vi "Averager Compute with Image.vi"(8 "error in (no error)":errorcluster, 9 "Grayscale Image":T1, 10 "Data":dbl[](array[numeric]), 11 "Roughness Averager in":refnum<class "Roughness Averager.lvclass">) -> (0 "error out":errorcluster, 3 "Roughness Averager out":refnum<class "Roughness Averager.lvclass">)   [LabVIEW 2018, in "Roughness Averager.lvclass"]
uses:
  Roughness Averager.lvclass
  <vilib>/vision/Image Controls.llb/IMAQ Image.ctl
  Roughness Averager.lvclass/Roughness Averager.ctl
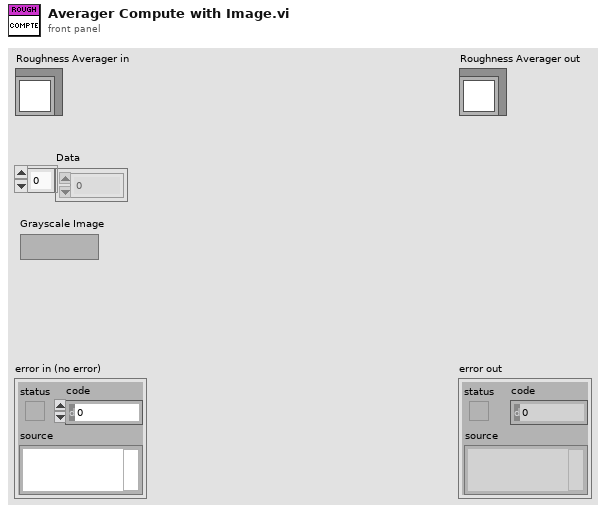
[diagram p1: front panel]
types:
  T1 = typedef "IMAQ Image.ctl" = refnum<image>
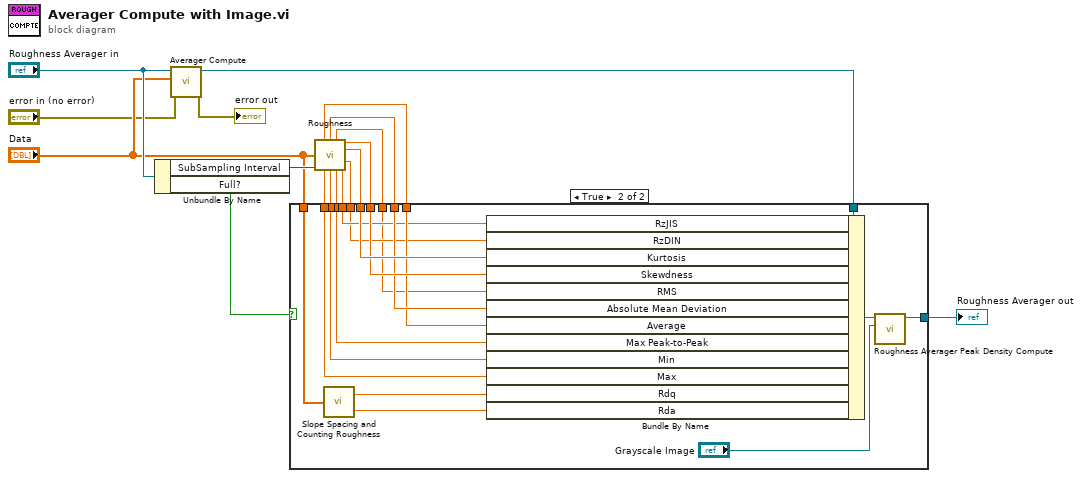
[diagram p0: block diagram]
diagram:
  n1 = Unbundle By Name("Roughness Averager in") -> ("SubSampling Interval"=w18:i32, "Full?"=w6:bool)
  n2 = call-dynamic "Averager Compute.vi"("error in (no error)"="error in (no error)", "Data"="Data", "Roughness Averager in"="Roughness Averager in") -> ("error out"=→"error out":errorcluster, "Roughness Averager out"=w1:refnum<class "Roughness Averager.lvclass">)  [unwired: 7 in]
  n3 = call "Roughness.vi"("Data"="Data", "Sub Sampling Interval (10)"=w18) -> ("Mean"=w14:dbl, "Absolute Mean Deviation"=w15:dbl, "RMS"=w8:dbl, "Skewdness"=w16:dbl, "Kurtosis"=w17:dbl, "RzDIN"=w9:dbl, "Max"=w11:dbl, "Min"=w12:dbl, "Max P-P"=w13:dbl, "RzJIS"=w10:dbl)  [unwired: 4 in]
  n4 = case shown="True" w6 {
    tunnel: w17 -> [_ w36]
    tunnel: w16 -> [_ w35]
    tunnel: w15 -> [_ w34]
    tunnel: w14 -> [_ w33]
    tunnel: w13 -> [_ w32]
    tunnel: w12 -> [_ w31]
    tunnel: w11 -> [_ w30]
    tunnel: w10 -> [_ w29]
    tunnel: w9 -> [_ w28]
    tunnel: w8 -> [_ w27]
    tunnel: "Data" -> [_ w26]
    tunnel: [w19 w23] -> w7
    tunnel: w1 -> [w19 w21]
    frame False {
    }
    frame True {
      n5 = call "Slope Spacing and Counting Roughness.vi"("Data"=w26) -> ("Rdq"=w25:dbl, "Rda"=w24:dbl)  [unwired: 4 in]
      n6 = Bundle By Name(cluster=w21, "RzJIS"=w29, "RzDIN"=w28, "Kurtosis"=w36, "Skewdness"=w35, "RMS"=w27, "Absolute Mean Deviation"=w34, "Average"=w33, "Max Peak-to-Peak"=w32, "Min"=w31, "Max"=w30, "Rdq"=w25, "Rda"=w24) -> (w20:refnum<class "Roughness Averager.lvclass">)
      n7 = call-dynamic "Roughness Averager Peak Density Compute.vi"("Grayscale Image"="Grayscale Image", "Roughness Averager in"=w20) -> ("Roughness Averager out"=w23:refnum<class "Roughness Averager.lvclass">)  [unwired: 8 in, 1 out]
    }
  }
  "Roughness Averager out" <- w7
